vi "JTMonitor.vi"() -> ()   [LabVIEW 2016]
uses:
  Utility/Monitor Communication/JT/JT-Status-DD.ctl
  Global/Global Variables/Data_Display_global.vi
panel:
  out "JT-Cluster":T1 {"Dump" scale=0.0..100.0}
  # "Dill. unit"
  # "LN2\nTrap"
  # "12"
  # "15"
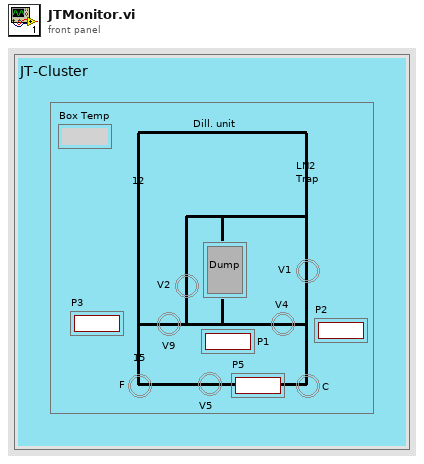
[diagram p1: front panel]
types:
  T1 = typedef "JT-Status-DD.ctl" = cluster{"V2":bool, "V5":bool, "V1":bool, "V9":bool, "F":bool, "C":bool, "V4":bool, "Dump":u8, "P3":dbl, "P1":dbl, "P2":dbl, "P5":dbl, "Box Temp":dbl}
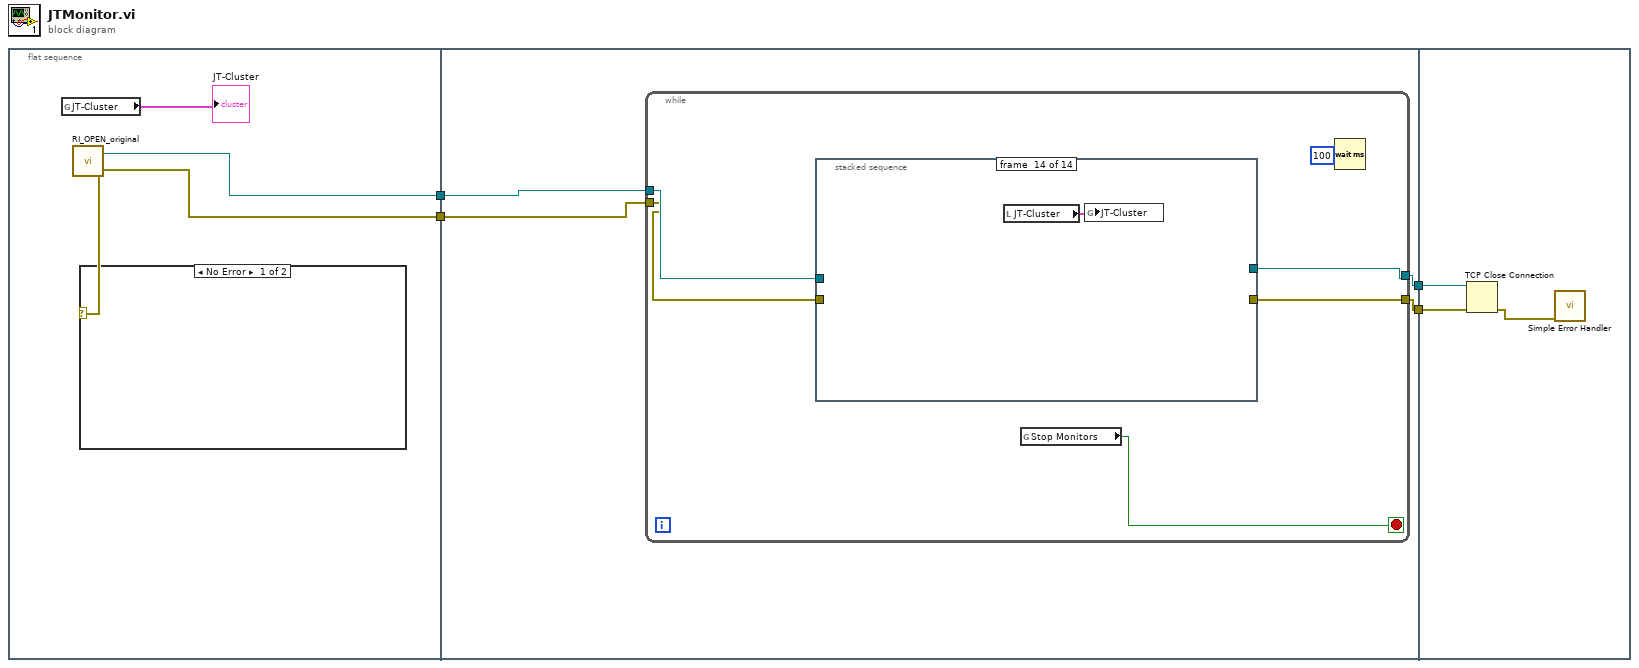
[diagram p0: block diagram]
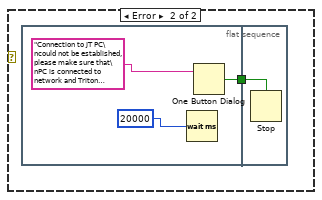
[diagram p2: hidden frame]
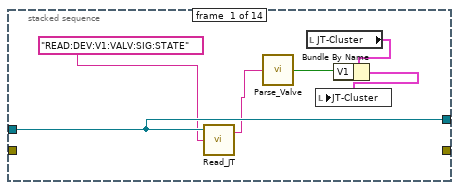
[diagram p3: hidden frame]
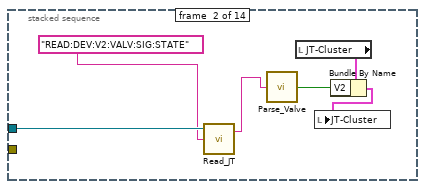
[diagram p4: hidden frame]
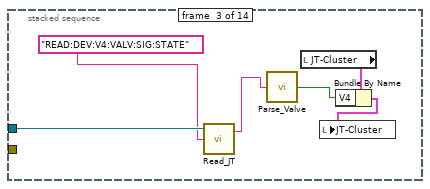
[diagram p5: hidden frame]
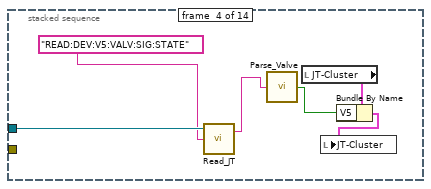
[diagram p6: hidden frame]
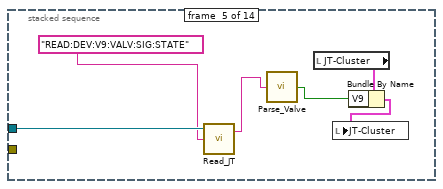
[diagram p7: hidden frame]
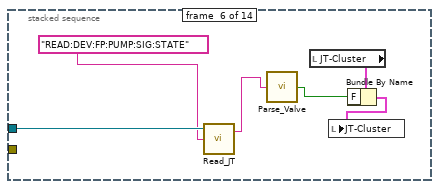
[diagram p8: hidden frame]
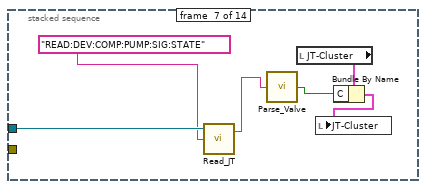
[diagram p9: hidden frame]
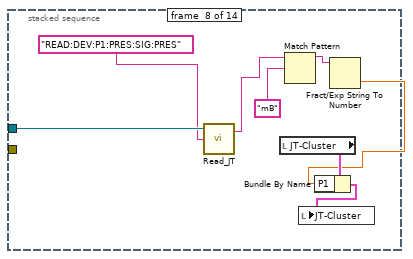
[diagram p10: hidden frame]
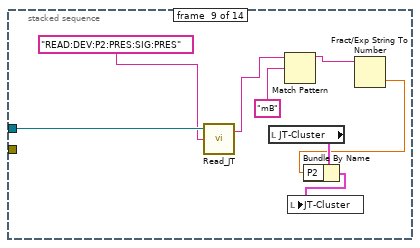
[diagram p11: hidden frame]
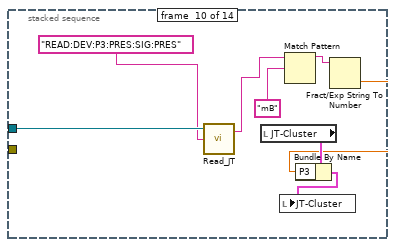
[diagram p12: hidden frame]
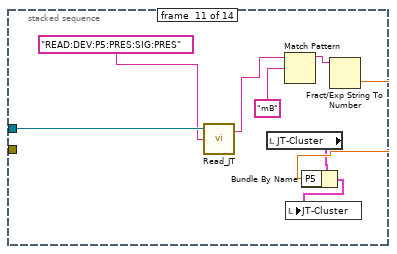
[diagram p13: hidden frame]
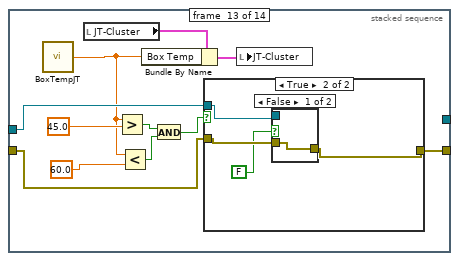
[diagram p15: hidden frame]
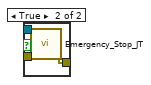
[diagram p17: hidden frame]
diagram:
  n1 = flat-sequence {
    tunnel: [w7] -> w2
    tunnel: [w6] -> w1
    tunnel: [w16] -> w4
    tunnel: [w15] -> w3
    tunnel: w2 -> [w14]
    tunnel: w1 -> [w13]
    tunnel: w4 -> [w119]
    tunnel: w3 -> [w118]
    frame #0 {
      n2 = global read "Data_Display_global.vi" "JT-Cluster"() -> (→"JT-Cluster":T1)
      n3 = call "RI_OPEN_original.vi"() -> ("error out"=w6:errorcluster, "connection ID"=w7:refnum<k5>)  [unwired: 3 in]
      n4 = case shown="No Error" w6 {
        frame No Error {
        }
        frame Error {
          n5 = flat-sequence {
            tunnel: [w9] -> w8
            tunnel: w8 -> [w12]
            frame #0 {
              n6 = Wait (ms)(milliseconds to wait=20000) -> ()  [unwired: 1 out]
              n7 = One Button Dialog(message="Connection to JT PC\ncould not be established, please make sure that\nPC is connected to network and Triton control software is running.\n\nThe JT monitor will be restarted in 20 seconds if the status monitor is not stopped meanwhile") -> (true=w9:bool)  [unwired: 1 in]
            }
            frame #1 {
              n8 = Stop(stop? (T)=w12) -> ()
            }
          }
        }
      }
    }
    frame #1 {
      n9 = while {
        tunnel: w14 -> [w21]
        tunnel: w13 -> [w19]
        tunnel: [w20] -> w16
        tunnel: [w17] -> w15
        stop <- w22 stop-if-true
        n10 = stacked-sequence {
          tunnel: w21 -> [w28 w34 w40 w46 w52 w58 w64 w72 w80 w88 w96 _ w103 _]
          tunnel: [w28 _ _ _ _ _ _ _ _ _ _ _ _ _] -> w20
          tunnel: w19 -> [_ _ _ _ _ _ _ _ _ _ _ _ w101 _]
          tunnel: [_ _ _ _ _ _ _ _ _ _ _ _ w102 _] -> w17
          frame #0 {
            n11 = call "Read_JT.vi"("Write"="READ:DEV:V1:VALV:SIG:STATE", "connection ID"=w28) -> ("Read"=w26:string)  [unwired: 1 in, 1 out]
            n12 = call "Parse_Valve.vi"("Valve"=w26) -> ("Status"=w23:bool)
            n13 = local read "JT-Cluster"() -> (w25:T1)
            n14 = Bundle By Name(cluster=w25, "V1"=w23) -> (w24:T1)
            n15 = local write "JT-Cluster"(w24) -> ()
          }
          frame #1 {
            n16 = call "Read_JT.vi"("Write"="READ:DEV:V2:VALV:SIG:STATE", "connection ID"=w34) -> ("Read"=w32:string)  [unwired: 1 in, 1 out]
            n17 = call "Parse_Valve.vi"("Valve"=w32) -> ("Status"=w29:bool)
            n18 = local read "JT-Cluster"() -> (w31:T1)
            n19 = Bundle By Name(cluster=w31, "V2"=w29) -> (w30:T1)
            n20 = local write "JT-Cluster"(w30) -> ()
          }
          frame #2 {
            n21 = call "Read_JT.vi"("Write"="READ:DEV:V4:VALV:SIG:STATE", "connection ID"=w40) -> ("Read"=w38:string)  [unwired: 1 in, 1 out]
            n22 = call "Parse_Valve.vi"("Valve"=w38) -> ("Status"=w35:bool)
            n23 = local read "JT-Cluster"() -> (w37:T1)
            n24 = Bundle By Name(cluster=w37, "V4"=w35) -> (w36:T1)
            n25 = local write "JT-Cluster"(w36) -> ()
          }
          frame #3 {
            n26 = call "Read_JT.vi"("Write"="READ:DEV:V5:VALV:SIG:STATE", "connection ID"=w46) -> ("Read"=w44:string)  [unwired: 1 in, 1 out]
            n27 = call "Parse_Valve.vi"("Valve"=w44) -> ("Status"=w41:bool)
            n28 = local read "JT-Cluster"() -> (w43:T1)
            n29 = Bundle By Name(cluster=w43, "V5"=w41) -> (w42:T1)
            n30 = local write "JT-Cluster"(w42) -> ()
          }
          frame #4 {
            n31 = call "Read_JT.vi"("Write"="READ:DEV:V9:VALV:SIG:STATE", "connection ID"=w52) -> ("Read"=w50:string)  [unwired: 1 in, 1 out]
            n32 = call "Parse_Valve.vi"("Valve"=w50) -> ("Status"=w47:bool)
            n33 = local read "JT-Cluster"() -> (w49:T1)
            n34 = Bundle By Name(cluster=w49, "V9"=w47) -> (w48:T1)
            n35 = local write "JT-Cluster"(w48) -> ()
          }
          frame #5 {
            n36 = call "Read_JT.vi"("Write"="READ:DEV:FP:PUMP:SIG:STATE", "connection ID"=w58) -> ("Read"=w56:string)  [unwired: 1 in, 1 out]
            n37 = call "Parse_Valve.vi"("Valve"=w56) -> ("Status"=w53:bool)
            n38 = local read "JT-Cluster"() -> (w55:T1)
            n39 = Bundle By Name(cluster=w55, "F"=w53) -> (w54:T1)
            n40 = local write "JT-Cluster"(w54) -> ()
          }
          frame #6 {
            n41 = call "Read_JT.vi"("Write"="READ:DEV:COMP:PUMP:SIG:STATE", "connection ID"=w64) -> ("Read"=w62:string)  [unwired: 1 in, 1 out]
            n42 = call "Parse_Valve.vi"("Valve"=w62) -> ("Status"=w59:bool)
            n43 = local read "JT-Cluster"() -> (w61:T1)
            n44 = Bundle By Name(cluster=w61, "C"=w59) -> (w60:T1)
            n45 = local write "JT-Cluster"(w60) -> ()
          }
          frame #7 {
            n46 = call "Read_JT.vi"("Write"="READ:DEV:P1:PRES:SIG:PRES", "connection ID"=w72) -> ("Read"=w70:string)  [unwired: 1 in, 1 out]
            n47 = local read "JT-Cluster"() -> (w67:T1)
            n48 = Match Pattern(string=w70, regular expression="mB") -> (before substring=w68:string)  [unwired: 1 in, 3 out]
            n49 = Fract/Exp String To Number(string=w68) -> (number=w65:dbl)  [unwired: 3 in, 1 out]
            n50 = Bundle By Name(cluster=w67, "P1"=w65) -> (w66:T1)
            n51 = local write "JT-Cluster"(w66) -> ()
          }
          frame #8 {
            n52 = call "Read_JT.vi"("Write"="READ:DEV:P2:PRES:SIG:PRES", "connection ID"=w80) -> ("Read"=w78:string)  [unwired: 1 in, 1 out]
            n53 = local read "JT-Cluster"() -> (w75:T1)
            n54 = Match Pattern(string=w78, regular expression="mB") -> (before substring=w76:string)  [unwired: 1 in, 3 out]
            n55 = Fract/Exp String To Number(string=w76) -> (number=w73:dbl)  [unwired: 3 in, 1 out]
            n56 = Bundle By Name(cluster=w75, "P2"=w73) -> (w74:T1)
            n57 = local write "JT-Cluster"(w74) -> ()
          }
          frame #9 {
            n58 = call "Read_JT.vi"("Write"="READ:DEV:P3:PRES:SIG:PRES", "connection ID"=w88) -> ("Read"=w86:string)  [unwired: 1 in, 1 out]
            n59 = local read "JT-Cluster"() -> (w83:T1)
            n60 = Match Pattern(string=w86, regular expression="mB") -> (before substring=w84:string)  [unwired: 1 in, 3 out]
            n61 = Fract/Exp String To Number(string=w84) -> (number=w81:dbl)  [unwired: 3 in, 1 out]
            n62 = Bundle By Name(cluster=w83, "P3"=w81) -> (w82:T1)
            n63 = local write "JT-Cluster"(w82) -> ()
          }
          frame #10 {
            n64 = call "Read_JT.vi"("Write"="READ:DEV:P5:PRES:SIG:PRES", "connection ID"=w96) -> ("Read"=w94:string)  [unwired: 1 in, 1 out]
            n65 = local read "JT-Cluster"() -> (w89:T1)
            n66 = Match Pattern(string=w94, regular expression="mB") -> (before substring=w92:string)  [unwired: 1 in, 3 out]
            n67 = Fract/Exp String To Number(string=w92) -> (number=w90:dbl)  [unwired: 3 in, 1 out]
            n68 = Bundle By Name(cluster=w89, "P5"=w90) -> (w91:T1)
            n69 = local write "JT-Cluster"(w91) -> ()
          }
          frame #11 {
          }
          frame #12 {
            n70 = call "BoxTempJT.vi"() -> ("Box Temperature"=w97:dbl)
            n71 = local read "JT-Cluster"() -> (w99:T1)
            n72 = Greater?(x=w97, y=45.0) -> (0:w106:bool)
            n73 = Less?(x=w97, y=60.0) -> (x < y?=w105:bool)
            n74 = Bundle By Name(cluster=w99, "Box Temp"=w97) -> (w98:T1)
            n75 = And(x=w106, y=w105) -> (x .and. y?=w104:bool)
            n76 = case shown="True" w104 {
              tunnel: w103 -> [_ w112]
              tunnel: w101 -> [w108 w111]
              tunnel: [w108 w110] -> w102
              frame False {
              }
              frame True {
                n77 = case shown="False" FALSE {
                  tunnel: w112 -> [_ w116]
                  tunnel: w111 -> [w113 w115]
                  tunnel: [w113 w114] -> w110
                  frame False {
                  }
                  frame True {
                    n78 = call "Emergency_Stop_JT.vi"("error in"=w115, "connection ID"=w116) -> ("error out"=w114:errorcluster)  [unwired: 9 in]
                  }
                }
              }
            }
            n79 = local write "JT-Cluster"(w98) -> ()
          }
          frame #13 {
            n80 = local read "JT-Cluster"() -> (w117:T1)
            n81 = global write "Data_Display_global.vi" "JT-Cluster"(w117) -> ()
          }
        }
        n82 = global read "Data_Display_global.vi" "Stop Monitors"() -> (w22:bool)
        n83 = Wait (ms)(milliseconds to wait=100) -> ()  [unwired: 1 out]
      }
    }
    frame #2 {
      n84 = TCP Close Connection(connection ID=w119, error in (no error)=w118) -> (error out=w120:errorcluster)  [unwired: 1 in, 1 out]
      n85 = call <vilib>:"Simple Error Handler.vi"("error in (no error)"=w120) -> ()  [unwired: 4 in, 5 out]
    }
  }
